vi "Init Active Devices.vi"(8 "error in":errorcluster, 10 "Device Names":string, 11 "DAC TC Temperature in":refnum<class "DAC TC Temp CryoSep.lvclass">) -> (0 "error out":errorcluster, 3 "DAC TC Temperature out":refnum<class "DAC TC Temp CryoSep.lvclass">)   [LabVIEW 2019, in "DAC.lvlib" / "DAC TC Temp CryoSep.lvclass"]
uses:
  DAC TC Temp CryoSep.lvclass
  C:/Users/krio/Documents/LV_Projects/test-stand/App/DAC/DAC.lvclass
  DAC.lvclass/DAC.ctl
  DAC TC Temp CryoSep.lvclass/DAC TC Temp CryoSep.ctl
  DAC.lvclass
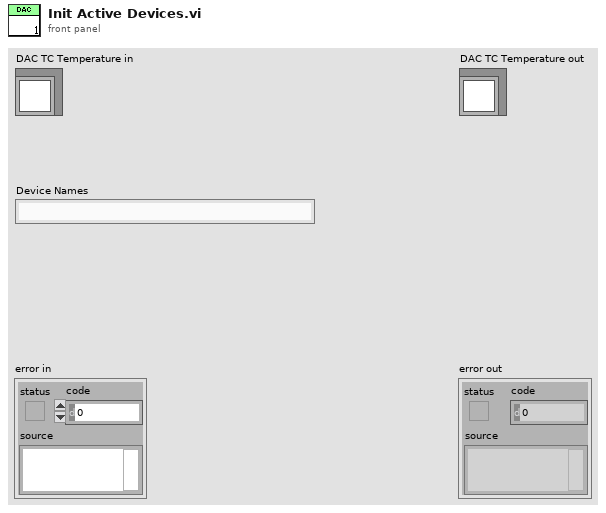
[diagram p1: front panel]
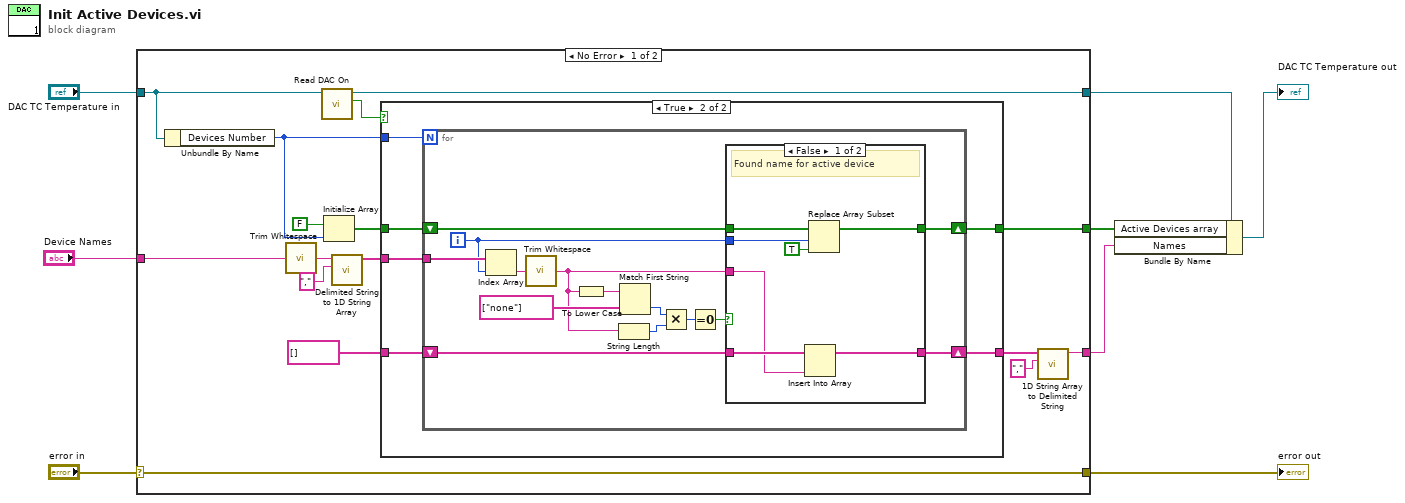
[diagram p0: block diagram]
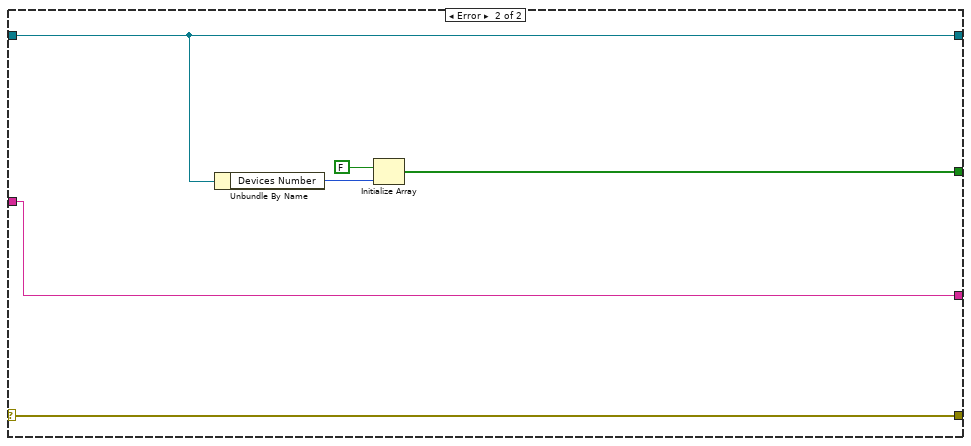
[diagram p4: hidden frame]
diagram:
  n1 = case shown="No Error" "error in" {
    selector: "error in" -> [w17 w61]
    tunnel: [w17 w61] -> w7
    tunnel: [w15 w58] -> w5
    tunnel: "DAC TC Temperature in" -> [w16 w58]
    tunnel: [w18 w57] -> w2
    tunnel: "Device Names" -> [w13 w56]
    tunnel: [w9 w56] -> w1
    frame No Error {
      n2 = Unbundle By Name(w16) -> ("Devices Number"=w20:i32)
      n3 = call <vilib>:"Trim Whitespace.vi"("string"=w13) -> ("trimmed string"=w24:string)  [unwired: 1 in]
      n4 = call "Read DAC On.vi"("DAC in"=w16) -> ("DAC On"=w14:bool, "DAC out"=w15:refnum<class "DAC TC Temp CryoSep.lvclass">)  [unwired: 8 in, 1 out]
      n5 = Initialize Array(FALSE, w20) -> (w19:bool[])
      n6 = call <vilib>:"Delimited String to 1D String Array.vi"("delimiter"=",", "delimited string"=w24) -> ("string array"=w21:string[])  [unwired: 9 in]
      n7 = case shown="True" w14 {
        tunnel: w21 -> [w25 w32]
        tunnel: w20 -> [_ w31]
        tunnel: w19 -> [w26 w30]
        tunnel: [w26 w29] -> w18
        tunnel: string[] [] -> [_ w28]
        tunnel: [w25 w27] -> w11
        frame False {
        }
        frame True {
          n8 = for {
            N: w31 -> [_]
            tunnel: w32 -> [w46]
            shift-right: [w37] -> w29
            shift-left: w30 -> [w38]
            shift-right: [w35] -> w27
            shift-left: w28 -> [w36]
            i -> [w39]
            n9 = Index Array(array=w46, index=w39) -> (element=w45:string)
            n10 = call <vilib>:"Trim Whitespace.vi"("string"=w45) -> ("trimmed string"=w33:string)  [unwired: 1 in]
            n11 = To Lower Case(string=w33) -> (all lower case string=w34:string)
            n12 = String Length(string=w33) -> (length=w43:i32)
            n13 = Match First String(2:string[] ["none"], 3:w34) -> (0:w42:i32)  [unwired: 1 out]
            n14 = Multiply(x=w42, y=w43) -> (x*y=w41:i32)
            n15 = Equal To 0?(x=w41) -> (x = 0?=w40:bool)
            n16 = case shown="False" w40 {
              tunnel: w33 -> [w48 _]
              tunnel: w39 -> [w52 _]
              tunnel: w38 -> [w53 w55]
              tunnel: [w50 w55] -> w37
              tunnel: w36 -> [w49 w54]
              tunnel: [w47 w54] -> w35
              frame False {
                # "Found name for active device"
                n17 = Insert Into Array "Insert Into Array"(array=w49, new element=w48) -> (w47:string[])  [unwired: 1 in]
                n18 = Replace Array Subset "Replace Array Subset"(array=w53, new element=TRUE ("new element/subarray"), index=w52) -> (w50:bool[])
              }
              frame True {
                # "Empty or 'none' - inactive device"
              }
            }
          }
        }
      }
      n19 = call <vilib>:"1D String Array to Delimited String.vi"("delimiter"=",", "string array"=w11) -> ("delimited string"=w9:string)  [unwired: 9 in]
    }
    frame Error {
      n20 = Unbundle By Name(w58) -> ("Devices Number"=w59:i32)
      n21 = Initialize Array(FALSE, w59) -> (w57:bool[])
    }
  }
  "error out" <- w7
  n22 = Bundle By Name(cluster=w5, "Active Devices array"=w2, "Names"=w1) -> (→"DAC TC Temperature out":refnum<class "DAC TC Temp CryoSep.lvclass">)
